vi "Send.vi"(8 "error in (no error)":errorcluster, 10 "Data":refnum<class "Data.lvclass">, 11 "ENET in":refnum<class "ENET_BS120x.lvclass">) -> (0 "error out":errorcluster, 3 "ENET out":refnum<class "ENET_BS120x.lvclass">)   [LabVIEW 2021, in "BS120x Driver.lvlib" / "ENET_BS120x.lvclass"]
uses:
  ENET_BS120x.lvclass
  _Private/Data Classes/Data Class/Data.lvclass
  ENET_BS120x.lvclass/ENET_BS120x.ctl
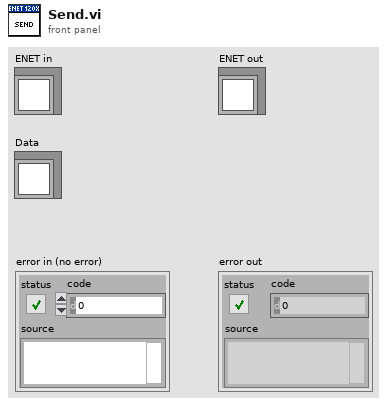
[diagram p1: front panel]
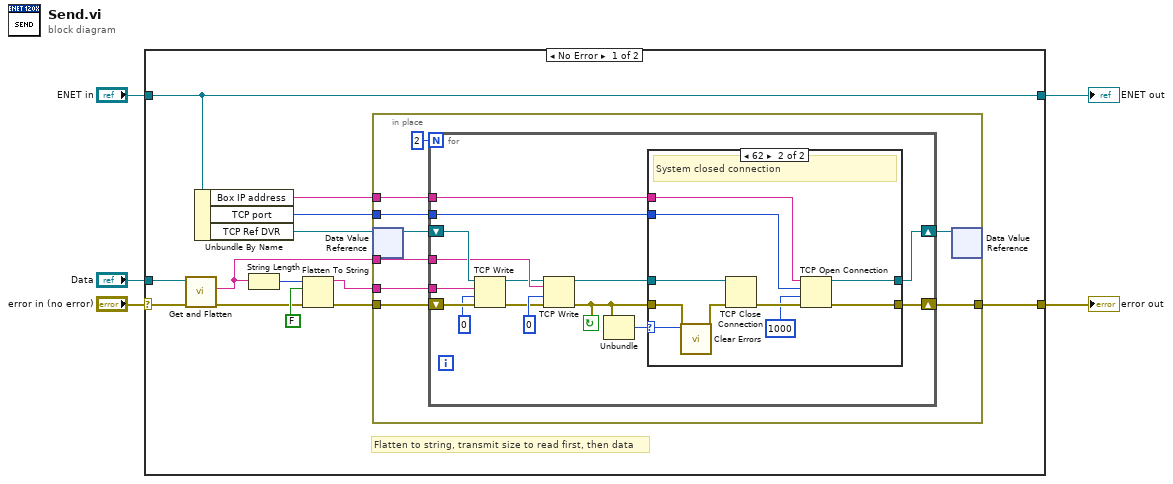
[diagram p0: block diagram]
diagram:
  n1 = case shown="No Error" "error in (no error)" {
    selector: "error in (no error)" -> [w10 w56]
    tunnel: [w8 w55] -> w5
    tunnel: "Data" -> [w18 _]
    tunnel: "ENET in" -> [w8 w55]
    tunnel: [w11 w56] -> w2
    frame No Error {
      # "Flatten to string, transmit size to read first, then data"
      n2 = call-dynamic "Get and Flatten.vi"("error in (no error)"=w10, "Data in"=w18) -> ("error out"=w12:errorcluster, "Flattened data string"=w13:string)  [unwired: 7 in, 1 out]
      n3 = Unbundle By Name(w8) -> ("Box IP address"=w7:string, "TCP port"=w6:u16, "TCP Ref DVR"=w9:refnum<data-value>)
      n4 = String Length(string=w13) -> (length=w17:i32)
      n5 = Flatten To String(anything=w17, prepend array or string size? (T)=FALSE, error in (no error)=w12) -> (data string=w16:string, error out=w15:errorcluster)  [unwired: 1 in, 1 out]
      n6 = in-place {
        in-place-border: w16 -> [w27]
        in-place-border: w15 -> [w26]
        in-place-border: w13 -> [w25]
        in-place-border: [w24] -> w11
        in-place-border: w7 -> [w20]
        in-place-border: w6 -> [w19]
        n7 = in-place-dvr #1(w9) -> (w22:refnum<k5>)  [unwired: 1 out]
        n8 = for {
          N: 2 -> [_]
          tunnel: w27 -> [w40]
          tunnel: w25 -> [w36]
          shift-right: [w33] -> w21
          shift-left: w22 -> [w42]
          shift-right: [w31] -> w24
          shift-left: w26 -> [w39]
          tunnel: w20 -> [w29]
          tunnel: w19 -> [w28]
          stop <- w30 continue-if-true
          n9 = TCP Write(connection ID=w42, data in=w40, error in (no error)=w39, 9:0 ("timeout ms (25000)")) -> (connection ID out=w35:refnum<k5>, error out=w38:errorcluster)  [unwired: 1 out]
          n10 = TCP Write(connection ID=w35, data in=w36, error in (no error)=w38, 9:0 ("timeout ms (25000)")) -> (connection ID out=w34:refnum<k5>, error out=w30:errorcluster)  [unwired: 1 out]
          n11 = Unbundle(w30) -> ("code"=w32:i32)  [unwired: 2 out]
          n12 = case shown="62" w32 {
            selector: w32 -> [_ w47]
            tunnel: w34 -> [w44 w54]
            tunnel: [w43 w51] -> w31
            tunnel: [w44 w50] -> w33
            tunnel: w30 -> [w43 w53]
            tunnel: w29 -> [_ w46]
            tunnel: w28 -> [_ w45]
            frame 0, Default {
            }
            frame 62 {
              # "System closed connection"
              n13 = call <vilib>:"Clear Errors.vi"("error in (no error)"=w53, "specific error code to clear (0: all)"=w47) -> ("error out"=w48:errorcluster)  [unwired: 4 in, 1 out]
              n14 = TCP Close Connection(connection ID=w54, error in (no error)=w48) -> (error out=w52:errorcluster)  [unwired: 1 in, 1 out]
              n15 = TCP Open Connection(address=w46, remote port or service name=w45, timeout ms (60000)=1000 ("timeout ms (25000)"), error in (no error)=w52) -> (connection ID=w50:refnum<k5>, error out=w51:errorcluster)  [unwired: 1 in]
            }
          }
        }
        n16 = in-place-dvr #1(w21) -> ()  [unwired: 2 out]
      }
    }
    frame Error {
    }
  }
  "ENET out" <- w5
  "error out" <- w2
